vi "CreatePublicEvents.vi"(8 "error in (no error)":errorcluster, 11 "SMO.Example":refnum<class "SMO.Example.lvclass">) -> (0 "error out":errorcluster, 3 "SMO.Example out":refnum<class "SMO.Example.lvclass">)   [LabVIEW 2013, in "SMO.Example.lvclass"]
doc: "---------------------------------------------------------------\nJKI State Machine Objects™\nhttp://jki.net/state-machine-objects/\nCopyright (C) 2005-2015, JKI <info@jki.net>\nALL RIGHTS RESERVED"
uses:
  SMO.Example.lvclass
  Typedefs/DataChanged--EventData--Cluster.ctl
  src/SMO/SMO.lvclass
  SMO.Example.lvclass/SMO.Example.ctl
panel:
  # "For instructions on how to use the JKI State Machine Objects, examples and video tutorials, visit:\nhttp://jki.net/state-machine-objects/\n\nJKI State Machine Objects™\nhttp://jki.net/state-machine-objects/\nCopyright (C) 2005-2015, JKI <info@jki.net>\nALL RIGHTS RESERVED"
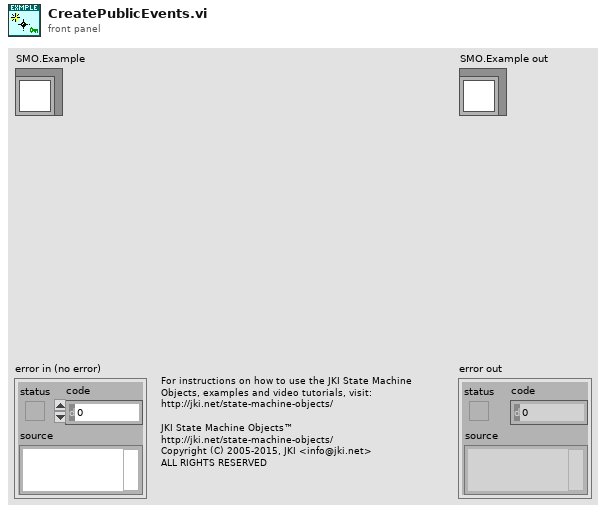
[diagram p1: front panel]
types:
  T1 = typedef "SMO.Example.lvclass/DataChanged--EventData--Cluster.ctl" = cluster{"Timestamp":timestamp, "Flow 1":dbl, "Flow 2":dbl}
  T2 = typedef "SMO.Example.lvclass/PrivateData--Ref.ctl" = refnum<data-value>
  T3 = typedef "SMO.Example.lvclass/PrivateData--Cluster.ctl" = cluster{"Configuration":T4, "Public Events":T5, "Protected Events":T6, "Flow 1":dbl, "Flow 2":dbl}
  T4 = typedef "SMO.Example.lvclass/Configuration--Cluster.ctl" = cluster{"Suffix":string}
  T5 = typedef "SMO.Example.lvclass/PublicEvents--Cluster.ctl" = cluster{"Data Changed":refnum<user-event>, "State Changed":refnum<user-event>}
  T6 = typedef "SMO.Example.lvclass/ProtectedEvents--Cluster.ctl" = cluster{"API_Template":refnum<user-event>, "PumpState":refnum<user-event>, "Valve State":refnum<user-event>}
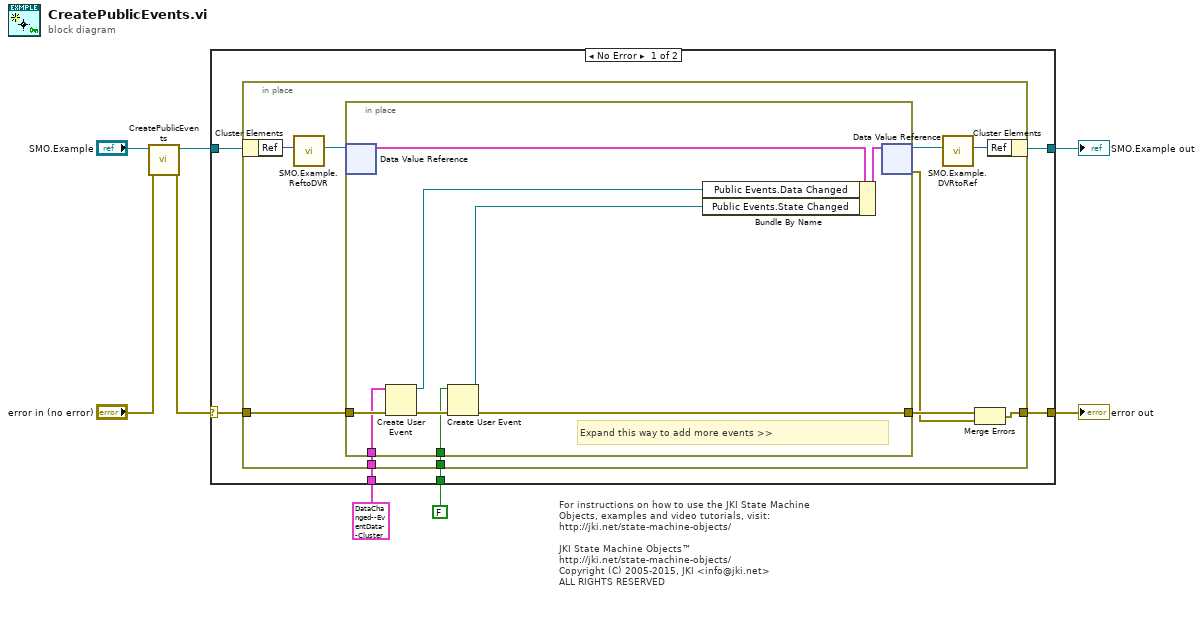
[diagram p0: block diagram]
diagram:
  # "For instructions on how to use the JKI State Machine Objects, examples and video tutorials, visit:\nhttp://jki.net/state-machine-objects/\n\nJKI State Machine Objects™\nhttp://jki.net/state-machine-objects/\nCopyright (C) 2005-2015, JKI <info@jki.net>\nALL RIGHTS RESERVED"
  n1 = call-parent "CreatePublicEvents.vi"("error in (no error)"="error in (no error)", "SMO"="SMO.Example") -> ("error out"=w2:errorcluster, "SMO out"=w4:refnum<class "SMO.Example.lvclass">)  [unwired: 8 in]
  n2 = case shown="No Error" w2 {
    selector: w2 -> [w12 w35]
    tunnel: [w11 w35] -> w7
    tunnel: [w13 w34] -> w8
    tunnel: w4 -> [w14 w34]
    tunnel: T1 {"Timestamp"=timestamp(0 s since 1904-01-01), "Flow 1"=0.0, "Flow 2"=0.0} ("Data In Event Data") -> [w10 _]
    tunnel: FALSE ("Pump State") -> [w9 _]
    frame No Error {
      n3 = in-place {
        in-place-border: w12 -> [w24]
        in-place-border: [w21] -> w11
        in-place-border: w10 -> [w20]
        in-place-border: w9 -> [w15]
        n4 = in-place-cluster #1(w14) -> ("Ref"=w19:u32)
        n5 = call "SMO.Example.ReftoDVR.vi"("Ref"=w19) -> ("Ref"=w18:T2)  [unwired: 10 in]
        n6 = in-place {
          in-place-border: w24 -> [w31]
          in-place-border: [w27] -> w23
          in-place-border: w20 -> [w30]
          in-place-border: w15 -> [w25]
          # "Expand this way to add more events >>"
          n7 = in-place-dvr #2(w18) -> (w32:T3)  [unwired: 1 out]
          n8 = Create User Event(user event datatype=w30, error in=w31) -> (user event=w29:refnum<user-event>, error out=w28:errorcluster)
          n9 = Create User Event(user event datatype=w25, error in=w28) -> (user event=w26:refnum<user-event>, error out=w27:errorcluster)
          n10 = Bundle By Name(cluster=w32, "Public Events.Data Changed"=w29, "Public Events.State Changed"=w26) -> (w33:T3)
          n11 = in-place-dvr #2(w33) -> (w17:T2, w22:errorcluster)
        }
        n12 = call "SMO.Example.DVRtoRef.vi"("Ref"=w17) -> ("Ref"=w16:u32)  [unwired: 10 in]
        n13 = Merge Errors(w23, w22) -> (w21:errorcluster)
        n14 = in-place-cluster #1("Ref"=w16) -> (w13:refnum<class "SMO.Example.lvclass">)
      }
    }
    frame Error {
    }
  }
  "error out" <- w7
  "SMO.Example out" <- w8
